vi "9.3.-SubVI Centroide de Imagen.vi"(9 "reference in":refnum<vi>, 10 "Array in":u32[][](array[numeric]), 11 "Digital in":refnum<vi>) -> (0 "y":dbl[](array[numeric]), 1 "Yc":dbl, 2 "Xc":dbl, 3 "row":i32, 4 "x":dbl[](array[numeric]), 5 "fx":dbl[](array[numeric]), 6 "col":i32, 7 "fy":dbl[](array[numeric]))   [LabVIEW 2020]
panel:
  # "Visión Artificial - Firma de Figuras\nDiego Cervantes Rodríguez\ndicer0.com"
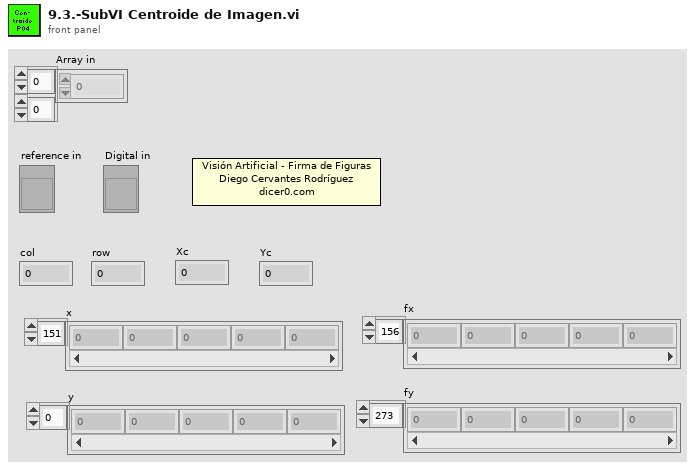
[diagram p1: front panel]
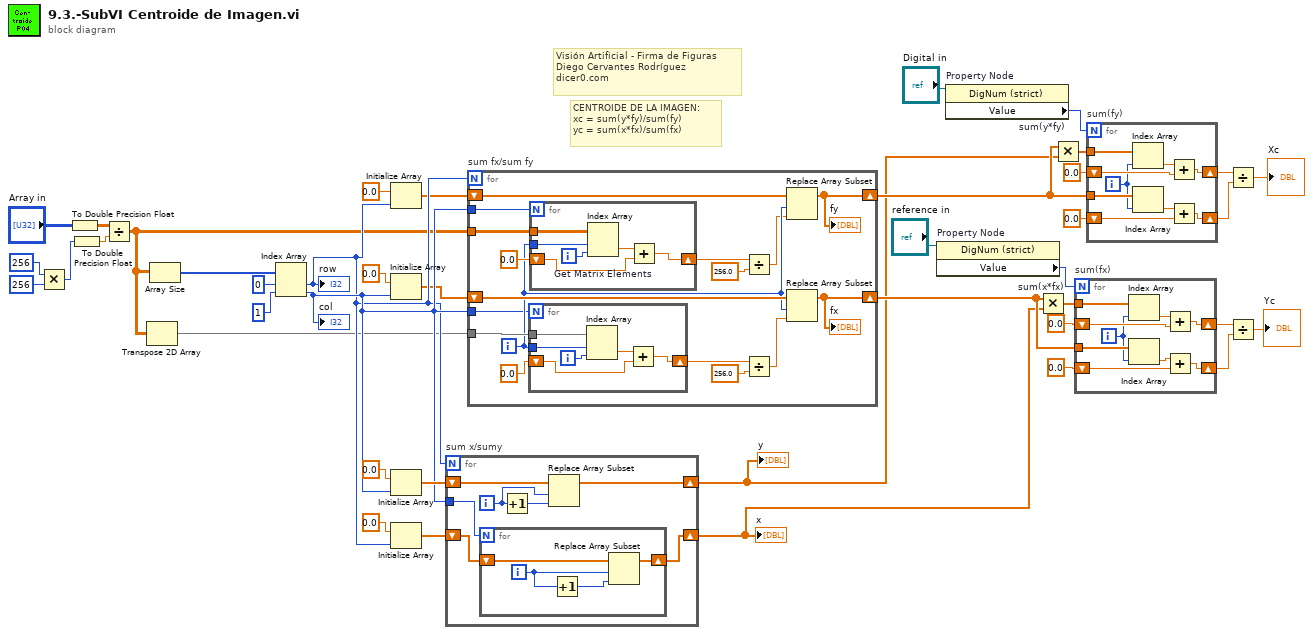
[diagram p0: block diagram]
diagram:
  # "Visión Artificial - Firma de Figuras\nDiego Cervantes Rodríguez\ndicer0.com"
  # "CENTROIDE DE LA IMAGEN:\nxc = sum(y*fy)/sum(fy)\nyc = sum(x*fx)/sum(fx)"
  n1 = Multiply(x=256, y=256) -> (x*y=w1:i32)
  n2 = To Double Precision Float(number="Array in") -> (double precision float=w3:dbl[][])
  n3 = To Double Precision Float(number=w1) -> (double precision float=w2:dbl)
  n4 = Divide(x=w3, y=w2) -> (x/y=w17:dbl[][])
  n5 = Transpose 2D Array(2D array=w17) -> (transposed array=w16:dbl[][])
  n6 = Array Size(array=w17) -> (size(s)=w9:i32[])
  n7 = Index Array "Index Array"(array=w9, index #1=0 ("index"), index #2=1 ("index")) -> (element #1=w20:i32, element #2=w21:i32)
  "col" <- w21
  "row" <- w20
  n8 = Initialize Array "Initialize Array"(0.0 ("element"), w20) -> (w12:dbl[])
  n9 = Initialize Array(0.0 ("element"), w21) -> (w15:dbl[])
  n10 = Initialize Array(0.0 ("element"), w21) -> (w22:dbl[])
  n11 = Initialize Array(0.0 ("element"), w20) -> (w23:dbl[])
  n12 = for "sum x/sumy" {
    N: w20 -> [_]
    tunnel: w21 -> [w46]
    shift-right: [w42] -> w37
    shift-left: w23 -> [w43]
    shift-right: [w44] -> w24
    shift-left: w22 -> [w45]
    i -> [w48]
    n13 = for {
      N: w46 -> [_]
      shift-right: [w49] -> w42
      shift-left: w43 -> [w50]
      i -> [w52]
      n14 = Increment(x=w52) -> (x+1=w51:i32)
      n15 = Replace Array Subset(array=w50, new element=w51, index=w52) -> (w49:dbl[])
    }
    n16 = Increment(x=w48) -> (x+1=w47:i32)
    n17 = Replace Array Subset(array=w45, new element=w47, index=w48) -> (w44:dbl[])
  }
  "x" <- w37
  "y" <- w24
  n18 = for "sum fx/sum fy" {
    N: w20 -> [_]
    shift-right: [w65] -> w28
    shift-left: w12 -> [w66]
    tunnel: w21 -> [w68]
    tunnel: w17 -> [w67]
    shift-right: [w63] -> w39
    shift-left: w15 -> [w64]
    tunnel: w16 -> [w61]
    tunnel: w21 -> [w59]
    i -> [w60]
    n19 = for {
      N: w59 -> [_]
      shift-right: [w74] -> w54
      shift-left: 0.0 -> [w75]
      tunnel: w61 -> [w73]
      tunnel: w60 -> [w71]
      i -> [w72]
      n20 = Index Array ("Get Matrix Elements")(array=w73, index (row)=w71, index (col)=w72) -> (element=w70:dbl)
      n21 = Add ("Add.vi")(x=w70, y=w75) -> (x+y=w74:dbl)
    }
    n22 = for {
      N: w68 -> [_]
      shift-right: [w76] -> w58
      shift-left: 0.0 -> [w81]
      tunnel: w60 -> [w78]
      tunnel: w67 -> [w80]
      i -> [w77]
      n23 = Index Array "Get Matrix Elements"(array=w80, index (row)=w78, index (col)=w77) -> (element=w79:dbl)
      n24 = Add ("Add.vi")(x=w79, y=w81) -> (x+y=w76:dbl)
    }
    n25 = Divide(x=w58, y=256.0) -> (x/y=w57:dbl)
    n26 = Divide(x=w54, y=256.0) -> (x/y=w53:dbl)
    n27 = Replace Array Subset(array=w66, new element=w57, index=w60) -> (w65:dbl[])
    "fy" <- w65
    n28 = Replace Array Subset(array=w64, new element=w53, index=w60) -> (w63:dbl[])
    "fx" <- w63
  }
  n29 = property on="Property Node" class="DigNum (strict)"(reference="reference in") -> ("Value"=w35:i32)  [unwired: 1 in, 2 out]
  n30 = property on="Property Node" class="DigNum (strict)"(reference="Digital in") -> ("Value"=w27:i32)  [unwired: 1 in, 2 out]
  n31 = Multiply "sum(x*fx)"(x=w39, y=w37) -> (x*y=w38:dbl[])
  n32 = Multiply "sum(y*fy)"(x=w28, y=w24) -> (x*y=w25:dbl[])
  n33 = for "sum(fx)" {
    N: w35 -> [_]
    tunnel: w38 -> [w90]
    shift-right: [w87] -> w33
    shift-left: 0.0 ("y") -> [w89]
    tunnel: w39 -> [w86]
    shift-right: [w82] -> w32
    shift-left: 0.0 ("y") -> [w83]
    i -> [w85]
    n34 = Index Array(array=w90, index=w85) -> (element=w88:dbl)
    n35 = Index Array(array=w86, index=w85) -> (element=w84:dbl)
    n36 = Add(x=w88, y=w89) -> (x+y=w87:dbl)
    n37 = Add(x=w84, y=w83) -> (x+y=w82:dbl)
  }
  n38 = for "sum(fy)" {
    N: w27 -> [_]
    tunnel: w25 -> [w99]
    shift-right: [w96] -> w30
    shift-left: 0.0 ("y") -> [w98]
    tunnel: w28 -> [w95]
    shift-right: [w91] -> w31
    shift-left: 0.0 ("y") -> [w92]
    i -> [w94]
    n39 = Index Array "Index Array"(array=w99, index=w94) -> (element=w97:dbl)
    n40 = Index Array(array=w95, index=w94) -> (element=w93:dbl)
    n41 = Add(x=w97, y=w98) -> (x+y=w96:dbl)
    n42 = Add(x=w93, y=w92) -> (x+y=w91:dbl)
  }
  n43 = Divide(x=w30, y=w31) -> (x/y=→"Xc":dbl)
  n44 = Divide(x=w33, y=w32) -> (x/y=→"Yc":dbl)
